vi "BRig_dataBlock_c_nTimeout_total.vi"() -> (2 "output_c_nTimeout_total":i32)   [LabVIEW 2014]
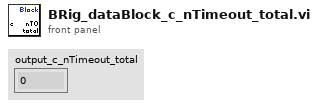
[diagram p1: front panel]
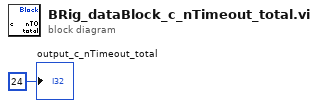
[diagram p0: block diagram]
diagram:
  "output_c_nTimeout_total" <- 24 ("output_iBlock")
